vi "Polling Core.vi"(8 "Error In":errorcluster, 11 "BNT_ULx-MCSV-DOPWM in":refnum<class "BNT_ULx-MCSV-DOPWM.lvclass">) -> (0 "Error Out":errorcluster, 3 "BNT_ULx-MCSV-DOPWM out":refnum<class "BNT_ULx-MCSV-DOPWM.lvclass">)   [LabVIEW 2021, in "BNT_ULx.lvlib" / "BNT_ULx-MCSV-DOPWM.lvclass"]
uses:
  BNT_ULx-MCSV-DOPWM.lvclass
  C:/Users/Holger/Documents/LVP/BNT/PGC/Packages/BNT_ULx/BNT_ULx-MCSV/BNT_ULx-MCSV.lvclass
  C:/Users/Holger/Documents/LVP/BNT/PGC/Packages/CSPP_Core/Actors/CSPP_BaseActor/CSPP_BaseActor.lvclass
  CSPP_Core/Actors/CSPP_BaseActor/CSPP_BaseActor.lvclass/CSPP_BaseActor.ctl
  BNT_ULx-MCSV-DOPWM.lvclass/BNT_ULx-MCSV-DOPWM.ctl
  <vilib>/Waveform/WDTOps.llb/WDT Get Waveform Subset DBL.vi
  <vilib>/Waveform/WDTOps.llb/WDT Get XY Value DBL.vi
  BNT_ULx-MCSV/BNT_ULx-MCSV.lvclass
  CSPP_Core/Actors/CSPP_BaseActor/CSPP_BaseActor.lvclass
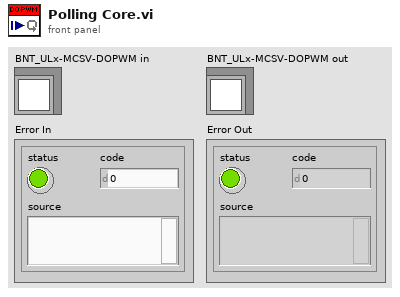
[diagram p1: front panel]
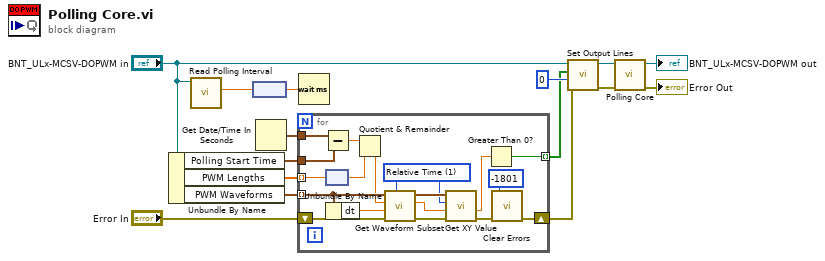
[diagram p0: block diagram]
diagram:
  n1 = Unbundle By Name("BNT_ULx-MCSV-DOPWM in") -> ("Polling Start Time"=w9:timestamp, "PWM Lengths"=w10:dbl[unit][], "PWM Waveforms"=w11:waveform(dbl)[])
  n2 = call "Read Polling Interval.vi"("CSPP_BaseActor in"="BNT_ULx-MCSV-DOPWM in") -> ("Polling Interval"=w8:dbl[unit])  [unwired: 8 in, 2 out]
  n3 = node(w8) -> (w7:dbl)
  n4 = Get Date/Time In Seconds() -> (seconds since 1Jan1904=w12:timestamp)
  n5 = for {
    tunnel: w11 -> [w33] mode=indexing
    shift-right: [w20] -> w4
    shift-left: "Error In" -> [w30]
    tunnel: [w23] -> w1 mode=indexing
    tunnel: w12 -> [w18]
    tunnel: w10 -> [w17] mode=indexing
    tunnel: w9 -> [w16]
    w25 = u16 1 items=["Samples", "Relative Time"] ("start/duration format")
    n6 = Subtract(x=w18, y=w16) -> (x-y=w32:dbl)
    n7 = node(w17) -> (w21:dbl)
    n8 = Unbundle By Name(w33) -> ("dt"=w31:dbl)
    n9 = Quotient & Remainder(x=w32, y=w21) -> (x-y*floor(x/y)=w22:dbl)  [unwired: 1 out]
    n10 = call-poly <vilib>:"Get Waveform Subset.vi"("start/duration format"=w25, "error in (no error)"=w30, "duration"=w31, "start samples/time"=w22, "waveform in"=w33) -> ("error out"=w28:errorcluster, "actual start samples/time"=w26:dbl, "waveform out"=w29:waveform(dbl))  [unwired: 1 in, 1 out]
    n11 = call-poly <vilib>:"Get XY Value.vi"("error in (no error)"=w28, "Y position"=w26, "Y position format"=w25, "waveform in"=w29) -> ("error out"=w27:errorcluster, "Y value"=w24:dbl)  [unwired: 3 in, 3 out]
    n12 = Greater Than 0?(x=w24) -> (x > 0?=w23:bool)
    n13 = call <vilib>:"Clear Errors.vi"("error in (no error)"=w27, "specific error code to clear (0: all)"=-1801) -> ("error out"=w20:errorcluster)  [unwired: 4 in, 1 out]
  }
  n14 = Wait (ms)(milliseconds to wait=w7) -> ()  [unwired: 1 out]
  n15 = call "Set Output Lines.vi"("Error In"=w4, "Start Index"=0, "DO Lines"=w1, "BNT_ULx-MCSV in"="BNT_ULx-MCSV-DOPWM in") -> ("Error Out"=w3:errorcluster, "BNT_ULx-MCSV out"=w5:refnum<class "BNT_ULx-MCSV-DOPWM.lvclass">)  [unwired: 6 in]
  n16 = call-parent "Polling Core.vi"("Error In"=w3, "BNT_ULx-MCSV in"=w5) -> ("Error Out"=→"Error Out":errorcluster, "BNT_ULx-MCSV out"=→"BNT_ULx-MCSV-DOPWM out":refnum<class "BNT_ULx-MCSV-DOPWM.lvclass">)  [unwired: 8 in]
